vi "display.vi"(8 "error in (no error)":errorcluster, 10 "GridRepresentable.lvclass":refnum<class "GridRepresentable.lvclass">, 11 "GridInputOutput in":refnum<class "GridInputOutput.lvclass">) -> (0 "error out":errorcluster, 3 "GridInputOutput out":refnum<class "GridInputOutput.lvclass">)   [LabVIEW 2020, in "GridInputOutput.lvclass"]
uses:
  GridInputOutput.lvclass
  GridDisplayable/GridRepresentable.lvclass
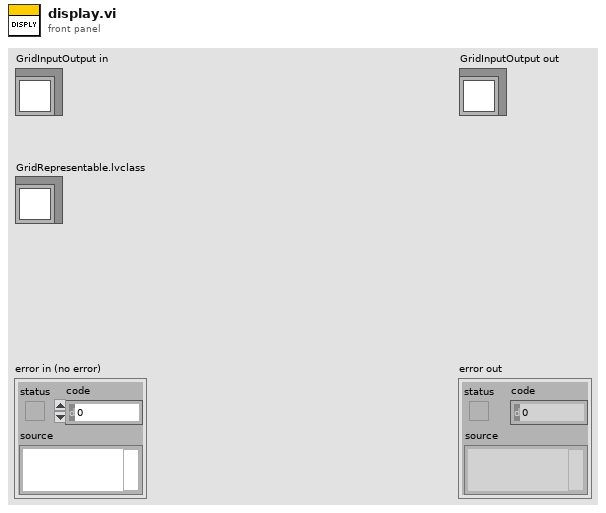
[diagram p1: front panel]
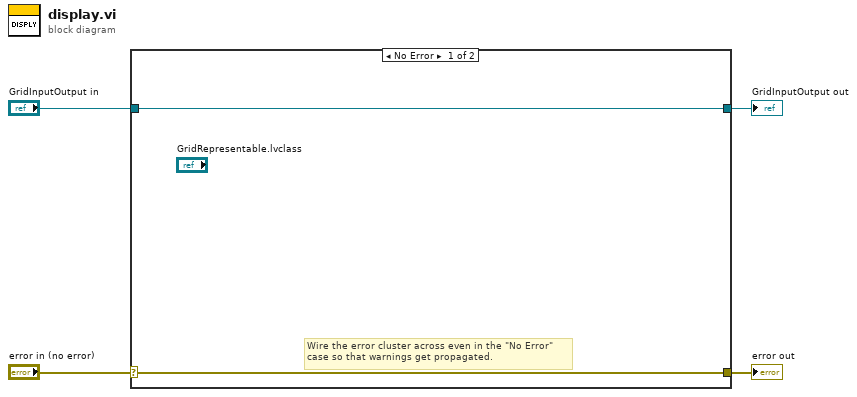
[diagram p0: block diagram]
diagram:
  n1 = case shown="No Error" "error in (no error)" {
    selector: "error in (no error)" -> [w5 w8]
    tunnel: [w5 w8] -> w3
    tunnel: [w6 w7] -> w1
    tunnel: "GridInputOutput in" -> [w6 w7]
    frame No Error {
      # "Wire the error cluster across even in the \"No Error\"\ncase so that warnings get propagated."
    }
    frame Error {
    }
  }
  "error out" <- w3
  "GridInputOutput out" <- w1
